vi "LI-U8 find base multiplier of A and B.vi"(3 "Large number - U8 B":T1, 5 "Large number - U8 A":T1) -> (0 "ratio of MSDs":u8, 1 "base multiplier":T1, 2 "Max # shifts (U8)":u8)   [LabVIEW 2012]
doc: "Finds the \"base multiplier\" of A and B . This is done by rounding A down so it only keeps highest digit (in base 256) and rounding B up in the same fashion, and dividing the two."
uses:
  User Access Type defs/Large number - U8 array.ctl
panel:
  # "index 0 = LSD"
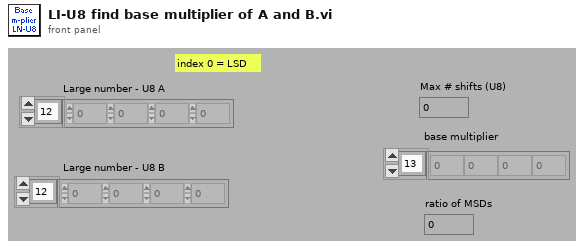
[diagram p1: front panel]
types:
  T1 = typedef "Large number - U8 array.ctl" = u8[]
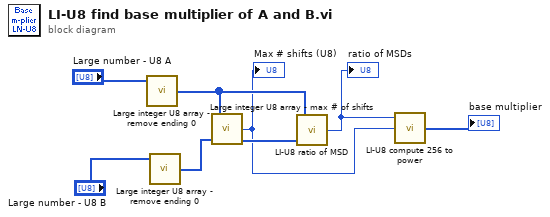
[diagram p0: block diagram]
diagram:
  n1 = call "Large integer U8 array - remove ending 0.vi"("Large number - U8"="Large number - U8 A") -> ("MSD zeros removed"=w5:T1)  [unwired: 4 out]
  n2 = call "Large integer U8 array - remove ending 0.vi"("Large number - U8"="Large number - U8 B") -> ("MSD zeros removed"=w6:T1)  [unwired: 4 out]
  n3 = call "Large integer U8 array - max # of shifts.vi"("LI-U8 B"=w6, "LI-U8 A"=w5) -> ("LI-U8 shifted B"=w4:T1, "Max # shifts (U8)"=w2:u8)  [unwired: 2 out]
  "Max # shifts (U8)" <- w2
  n4 = call "LI-U8 ratio of MSD.vi"("Large number - U8 B"=w4, "Large number - U8 A"=w5) -> ("ratio of MSDs"=w3:u8)  [unwired: 3 out]
  "ratio of MSDs" <- w3
  n5 = call "LI-U8 compute 256 to power.vi"("power (U32)"=w2, "X (U8)"=w3) -> ("x* 256^Power"=→"base multiplier":T1)  [unwired: 3 out]
